vi "GENser Write to Instrument.vi"(7 "GEN Addr":i16=-1, 8 "error":errorcluster, 10 "Command":string, 11 "VISA":refnum<visa-resource-name>="COM1") -> (0 "error out":errorcluster, 1 "Response":string, 3 "VISA out":refnum<visa-resource-name>)   [LabVIEW 2017]
doc: "This VI sends any Serial command to the GEN power supply. It verifies the response is \"OK\"\n\nThe Command cannot have a checksum. The checksum is added by the driver. A message terminator is optional. The driver will convert any terminator to a carriage return.\n\nThe \"GEN Address\" input is optional. If left unwired, the command will be sent to the address of the last instrument commanded.\n\nIfan error occurs and the command is rejected, the error message will be passed out of the \"error out\" cluster"
panel:
  # "Send Any Command"
  # "Lambda Genesys \n Serial Port\n  DC Power Supplies"
  # "Includes error checking.\nAdds checksum to cmd string"
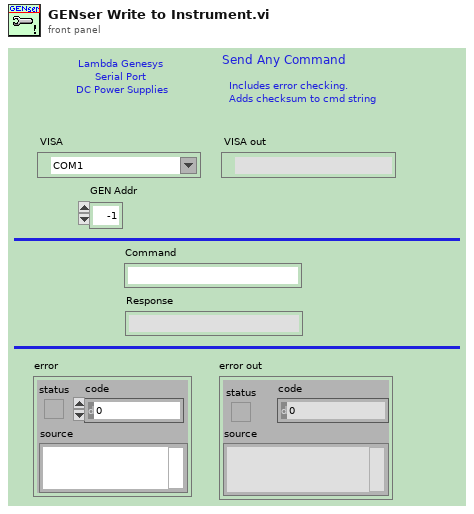
[diagram p1: front panel]
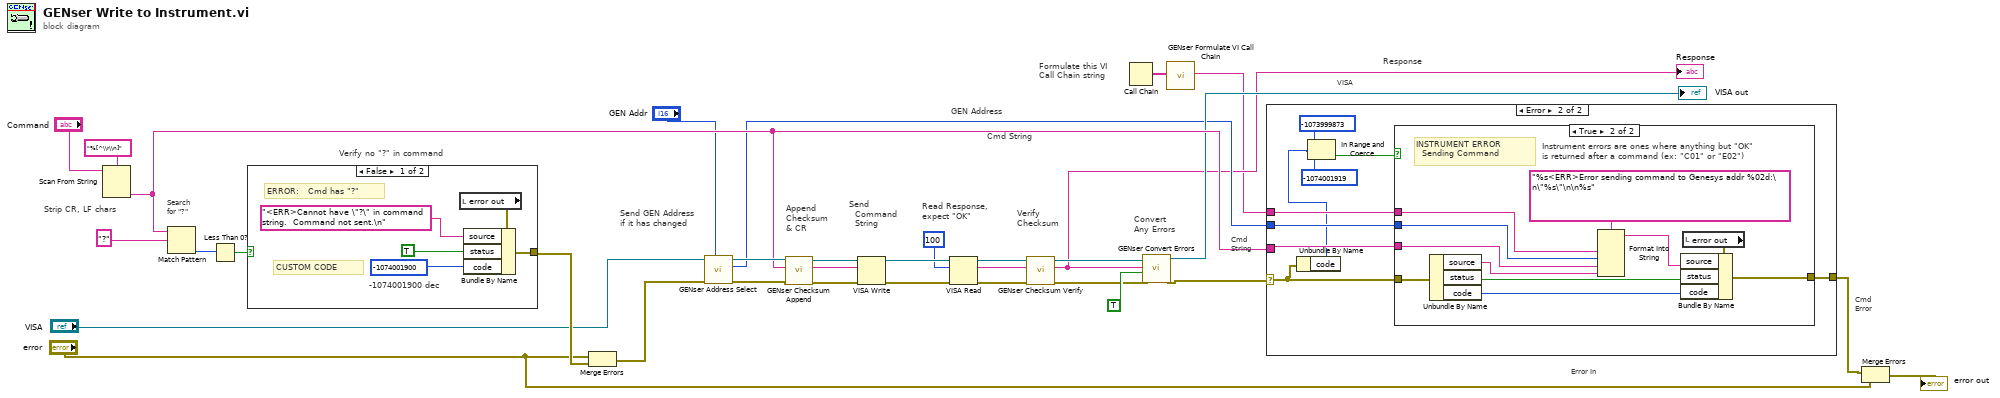
[diagram p0: block diagram]
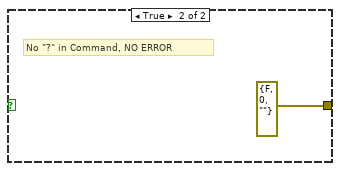
[diagram p2: hidden frame]
diagram:
  # "VISA"
  # "Response"
  # "GEN Address"
  # "Convert\nAny Errors"
  # "Verify\nChecksum"
  # "Append\nChecksum \n& CR"
  # "Cmd String"
  # "Cmd\nError"
  # "Error In"
  # "Cmd\nString"
  # "Verify no \"?\" in command"
  # "Send GEN Address\nif it has changed"
  # "Send  \n  Command  \n  String"
  # "Read Response,\nexpect \"OK\""
  # "Search\nfor \"?\""
  # "Strip CR, LF chars"
  # "Formulate this VI \nCall Chain string"
  n1 = Scan From String(format string="%[^\\r\\n]", input string="Command") -> (output 1=w14:string)  [unwired: 3 in, 3 out]
  n2 = Match Pattern(string=w14, regular expression="?") -> (offset past match=w30:i32)  [unwired: 1 in, 3 out]
  n3 = Less Than 0?(x=w30) -> (x < 0?=w31:bool)
  n4 = case shown="False" w31 {
    tunnel: [w35 errorcluster {"status"=FALSE, "code"=0, "source"=""} ("error out")] -> w28
    frame False {
      # "-1074001900 dec"
      # "CUSTOM CODE"
      # "ERROR:   Cmd has \"?\""
      n5 = local read "error out"() -> (w38:errorcluster)
      n6 = Bundle By Name(cluster=w38, "source"="<ERR>Cannot have \"?\" in command string.  Command not sent.\n" ("Source"), "status"=TRUE, "code"=-1074001900) -> (w35:errorcluster)
    }
    frame True {
      # "No \"?\" in Command, NO ERROR"
    }
  }
  n7 = Merge Errors("error", w28) -> (w23:errorcluster)
  n8 = call "GENser Address Select.vi"("GEN Addr"="GEN Addr", "error"=w23, "VISA"="VISA") -> ("error out"=w18:errorcluster, "Last GEN Addr"=w6:i16, "VISA out"=w19:refnum<visa-resource-name>)  [unwired: 6 in]
  n9 = call "GENser Checksum Append.vi"("error"=w18, "Input Cmd"=w14, "VISA"=w19) -> ("error out"=w16:errorcluster, "ChkSum Cmd"=w15:string, "VISA out"=w17:refnum<visa-resource-name>)  [unwired: 6 in]
  n10 = VISA Write(VISA resource name=w17, write buffer=w15, error in (no error)=w16) -> (VISA resource name out=w22:refnum<visa-resource-name>, error out=w21:errorcluster)  [unwired: 1 out]
  n11 = VISA Read(VISA resource name=w22, byte count=u32 100 ("byte count (0)"), error in (no error)=w21) -> (VISA resource name out=w13:refnum<visa-resource-name>, read buffer=w4:string, error out=w12:errorcluster)  [unwired: 1 out]
  n12 = call "GENser Checksum Verify.vi"("error"=w12, "String in"=w4, "VISA"=w13) -> ("error out"=w10:errorcluster, "Trimmed String"=w3:string, "VISA out"=w9:refnum<visa-resource-name>)  [unwired: 6 in]
  "Response" <- w3
  n13 = Call Chain() -> (call chain=w2:string[])
  n14 = call "GENser Convert Errors.vi"("error"=w10, "Expect \"OK\" (F)"=TRUE ("Expect \"OK\" (F)"), "String in"=w3, "VISA"=w9) -> ("error out"=w8:errorcluster, "VISA out"=→"VISA out":refnum<visa-resource-name>)  [unwired: 6 in]
  n15 = call "GENser Formulate VI Call Chain.vi"("Call Chain"=w2) -> ("String Out"=w1:string)  [unwired: 10 in]
  n16 = case shown="Error" w8 {
    selector: w8 -> [w40 w44]
    tunnel: w14 -> [_ w48]
    tunnel: [w40 w49] -> w26
    tunnel: w1 -> [_ w47]
    tunnel: w6 -> [_ w46]
    frame No Error {
      # "Command Sent Correctly \n  and \"OK\" Returned"
    }
    frame Error {
      n17 = Unbundle By Name(w44) -> ("code"=w43:i32)
      n18 = In Range and Coerce(upper limit=-1073999873 ("code"), x=w43, lower limit=-1074001919 ("code")) -> (In Range?=w45:bool)  [unwired: 1 out]
      n19 = case shown="True" w45 {
        tunnel: w44 -> [w50 w60]
        tunnel: [w50 w57] -> w49
        tunnel: w48 -> [_ w55]
        tunnel: w47 -> [_ w52]
        tunnel: w46 -> [_ w51]
        frame False {
          # "For VISA error, do not change error message"
          # "VISA  ERROR  \n  Sending Command"
        }
        frame True {
          # "Instrument errors are ones where anything but \"OK\"\nis returned after a command (ex: \"C01\" or \"E02\")"
          # "INSTRUMENT ERROR  \n  Sending Command"
          n20 = Unbundle By Name(w60) -> ("source"=w54:string, "status"=w58:bool, "code"=w59:i32)
          n21 = Format Into String(format string="%s<ERR>Error sending command to Genesys addr %02d:\n\"%s\"\n\n%s" ("Source"), w52, w51, w55, w54) -> (resulting string=w53:string)  [unwired: 2 in, 1 out]
          n22 = local read "error out"() -> (w61:errorcluster)
          n23 = Bundle By Name(cluster=w61, "source"=w53, "status"=w58, "code"=w59) -> (w57:errorcluster)
        }
      }
    }
  }
  n24 = Merge Errors("error", w26) -> (→"error out":errorcluster)
